vi "hw5_ques3.vi"() -> ()   [LabVIEW 2022 SP3]
uses:
  <vilib>/DAQmx/read.llb/DAQmx Read (Analog DBL 1Chan 1Samp).vi
  <vilib>/DAQmx/create/channels.llb/DAQmx Create Channel (AI-Voltage-Basic).vi
  <vilib>/DAQmx/configure/timing.llb/DAQmx Timing (Sample Clock).vi
  <vilib>/DAQmx/miscellaneous.llb/DAQmx Fill In Error Info.vi
panel:
  out "Waveform Chart 2":dbl(graph)
  out "Waveform Chart":dbl(graph)
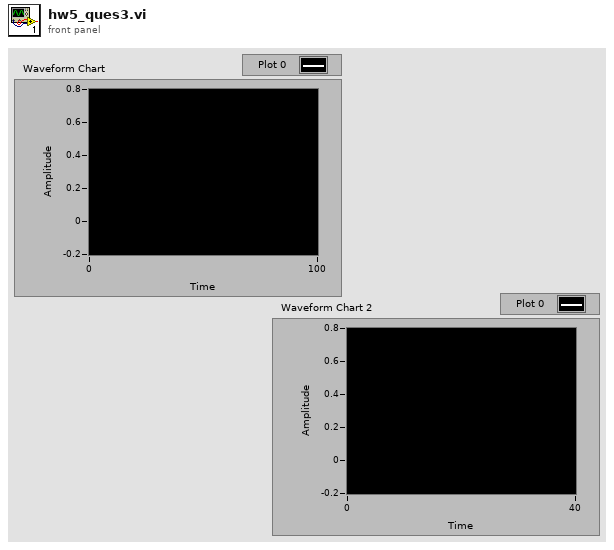
[diagram p1: front panel]
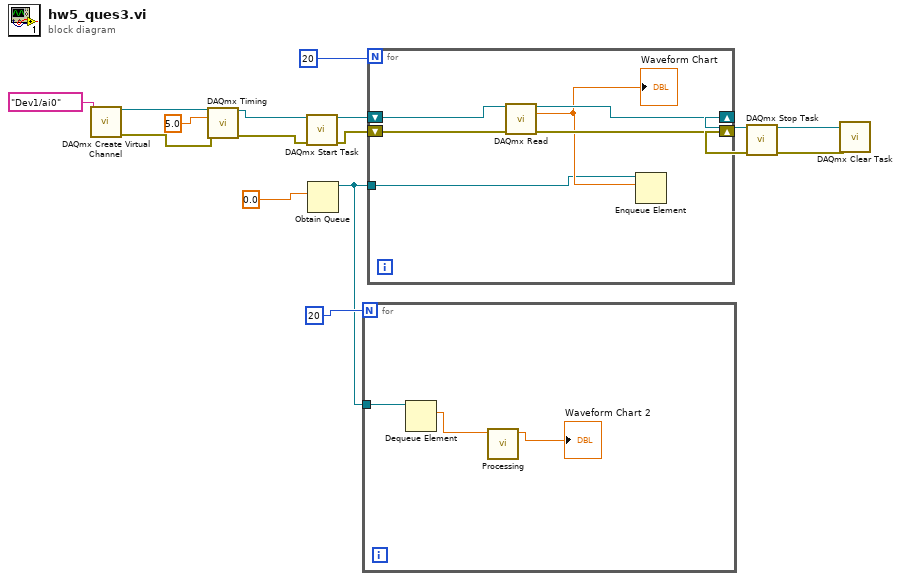
[diagram p0: block diagram]
diagram:
  n1 = call-poly <vilib>:"DAQmx Create Virtual Channel.vi"("physical channels"=tag "Dev1/ai0") -> ("task out"=w14:refnum<k21>, "error out"=w13:errorcluster)  [unwired: 13 in]
  n2 = call-poly <vilib>:"DAQmx Timing.vi"("task/channels in"=w14, "rate"=5.0, "error in"=w13) -> ("task out"=w11:refnum<k21>, "error out"=w12:errorcluster)  [unwired: 11 in]
  n3 = call <vilib>:"DAQmx Start Task.vi"("task/channels in"=w11, "error in"=w12) -> ("task out"=w10:refnum<k21>, "error out"=w9:errorcluster)  [unwired: 12 in]
  n4 = Obtain Queue(element data type=0.0) -> (queue out=w1:refnum<queue>)  [unwired: 4 in, 2 out]
  n5 = for {
    N: 20 -> [_]
    tunnel: w1 -> [w19]
    n6 = Dequeue Element(queue=w19) -> (element=w18:dbl)  [unwired: 2 in, 3 out]
    n7 = call "Processing.vi"("Input"=w18) -> ("Output"=→"Waveform Chart 2":dbl)  [unwired: 10 in]
  }
  n8 = for {
    N: 20 -> [_]
    shift-right: [w22] -> w8
    shift-left: w10 -> [w25]
    shift-right: [w23] -> w7
    shift-left: w9 -> [w24]
    tunnel: w1 -> [w20]
    n9 = call-poly <vilib>:"DAQmx Read.vi"("task/channels in"=w25, "error in"=w24) -> ("task out"=w22:refnum<k21>, "data"=w21:dbl, "error out"=w23:errorcluster)  [unwired: 11 in]
    "Waveform Chart" <- w21
    n10 = Enqueue Element(queue=w20, element=w21) -> ()  [unwired: 2 in, 3 out]
  }
  n11 = call <vilib>:"DAQmx Stop Task.vi"("task/channels in"=w8, "error in"=w7) -> ("task out"=w6:refnum<k21>, "error out"=w5:errorcluster)  [unwired: 12 in]
  n12 = call <vilib>:"DAQmx Clear Task.vi"("task in"=w6, "error in"=w5) -> ()  [unwired: 13 in, 1 out]
